vi "Edgertronic-download.vi"(3 "error in (no error)":errorcluster, 5 "URL":string="192.168.1.101") -> (0 "error out":errorcluster={"status"=FALSE, "code"=66, "source"="TCP Read in Edgertronic-GET_cmd.vi->Edgertronic-download.vi"}, 1 "Download":T1={"Download file extension"="/static/mnt/sdcard/DCIM/slomo_1465837839.mov", "Connection Information:"="HTTP/1.0 302 Found\r\nContent-Type: text/html; charset=utf-8\r\nContent-Length: 295\r\nLocation: http://0.0.0.0/static/mnt/sdcard/DCIM/slomo_1465837839.mov\r\nConnection: close\r\nDate: Tue, 14 Jun 2016 12:16:34 GMT\r\nServer: lighttpd/1.4.11 (edgertonic slow motion camera)"})   [LabVIEW 2015]
doc: "This VI downloads the last saved video marking data with MIME type video/quicktime."
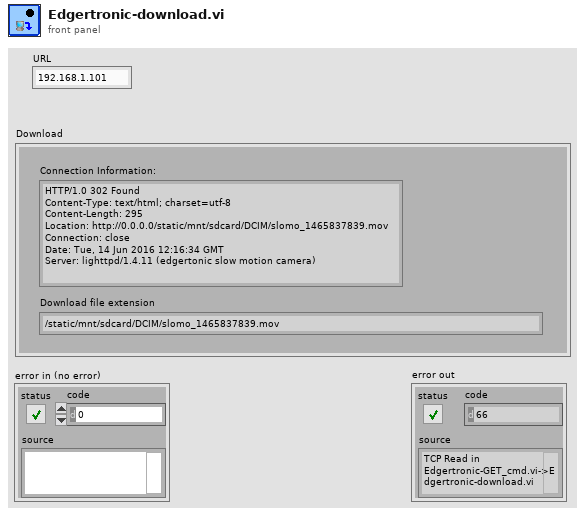
[diagram p1: front panel]
types:
  T1 = cluster{"Download file extension":string, "Connection Information:":string}
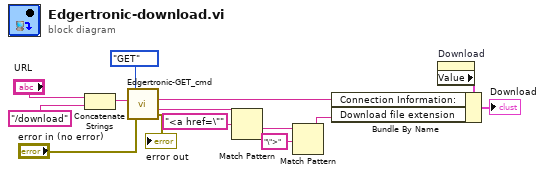
[diagram p0: block diagram]
diagram:
  n1 = Concatenate Strings("URL", "/download" ("GET Cmd")) -> (w2:string)
  n2 = call "Edgertronic-GET_cmd.vi"("error in (no error)"="error in (no error)", "URL"=w2, "Type"=enum16{"GET", "POST"}."GET") -> ("error out"=→"error out":errorcluster, "data"=w7:string, "Connection Info"=w8:string)  [unwired: 1 in]
  n3 = Match Pattern(string=w7, regular expression="<a href=\"") -> (after substring=w14:string)  [unwired: 1 in, 3 out]
  n4 = Match Pattern(string=w14, regular expression="\">") -> (before substring=w11:string)  [unwired: 1 in, 3 out]
  n5 = property on="Download" class="Clust (strict)"() -> ("Value"=w10:T1)  [unwired: 2 in, 2 out]
  n6 = Bundle By Name(cluster=w10, "Connection Information:"=w8, "Download file extension"=w11) -> (→"Download":T1)
